vi "write_log_path.vi"(8 "error in (no error)":errorcluster, 10 "log_path":path, 11 "data_logger in":refnum<class "data_logger.lvclass">) -> (0 "error out":errorcluster, 3 "data_logger out":refnum<class "data_logger.lvclass">)   [LabVIEW 2015, in "data_logger.lvclass"]
uses:
  data_logger.lvclass
  data_logger.lvclass/data_logger.ctl
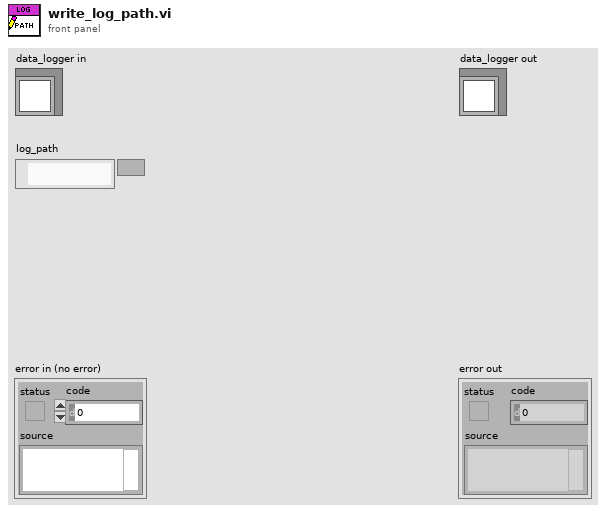
[diagram p1: front panel]
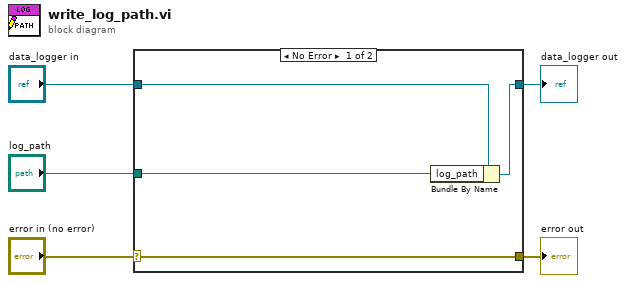
[diagram p0: block diagram]
diagram:
  n1 = case shown="No Error" "error in (no error)" {
    selector: "error in (no error)" -> [w9 w10]
    tunnel: [w9 w10] -> w4
    tunnel: [w7 w11] -> w2
    tunnel: "data_logger in" -> [w8 w11]
    tunnel: "log_path" -> [w6 _]
    frame No Error {
      n2 = Bundle By Name(cluster=w8, "log_path"=w6) -> (w7:refnum<class "data_logger.lvclass">)
    }
    frame Error {
    }
  }
  "error out" <- w4
  "data_logger out" <- w2
